vi "4 - Save a Well-Documented File (Solution).vi"() -> ()   [LabVIEW 2013]
uses:
  <vilib>/DAQmx/read.llb/DAQmx Read (Analog 1D Wfm NChan NSamp).vi
  <vilib>/DAQmx/miscellaneous.llb/DAQmx Fill In Error Info.vi
panel:
  out "Alarm Output":bool
  in  "Alarm Level":dbl=26.0
  out "Temperature":waveform(dbl)[](graph)
  in  "stop":bool
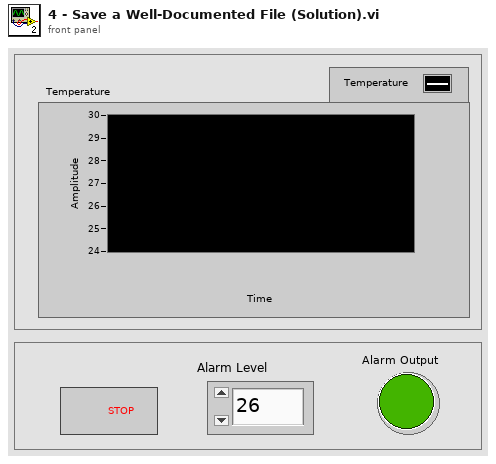
[diagram p1: front panel]
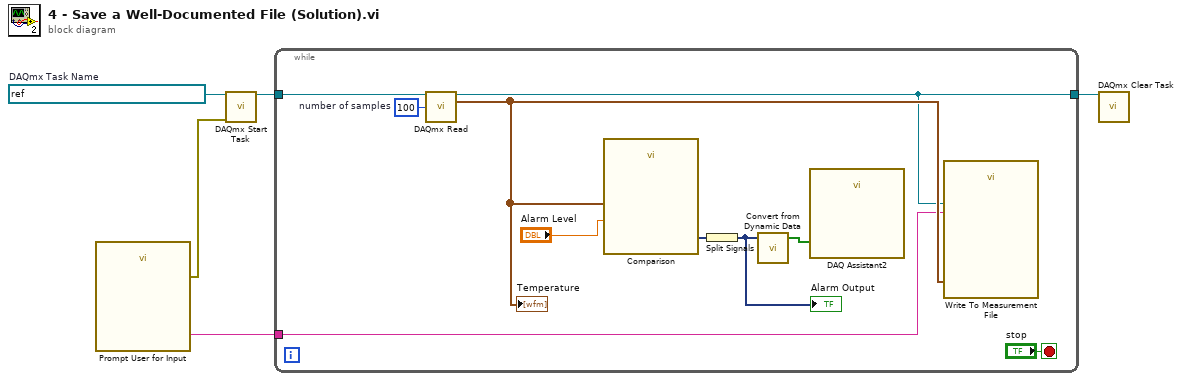
[diagram p0: block diagram]
diagram:
  w3 = refnum<k21> "Measure Temperature and Light"  # DAQmx Task Name
  n1 = call "Prompt User for Input"() -> ("Response"=w2:string, "error out"=w1:errorcluster)  [unwired: 17 in, 1 out]
  n2 = call <vilib>:"DAQmx Start Task.vi"("task/channels in"=w3, "error in"=w1) -> ("task out"=w5:refnum<k21>)  [unwired: 12 in, 1 out]
  n3 = while {
    tunnel: w5 -> [w11]
    tunnel: [w7] -> w4
    tunnel: w2 -> [w6]
    stop <- "stop" stop-if-true
    w9 = 100  # number of samples
    n4 = call-poly <vilib>:"DAQmx Read.vi"("task/channels in"=w11, "number of samples per channel"=w9) -> ("task out"=w7:refnum<k21>, "data"=w10:waveform(dbl)[])  [unwired: 11 in, 1 out]
    "Temperature" <- w10
    n5 = call "Comparison"("Operand 2"="Alarm Level", "Operand 1"=w10) -> ("Result"=w13:dynamicdata)  [unwired: 1 in, 8 out]
    n6 = Split Signals(w13) -> (w8:dynamicdata)  [unwired: 1 in]
    "Alarm Output" <- w8
    n7 = call "Convert from Dynamic Data"("Dynamic Data Type"=w8) -> ("Array"=w12:bool[])  [unwired: 3 in]
    n8 = call "DAQ Assistant2"("data"=w12) -> ()  [unwired: 4 in, 15 out]
    n9 = call "Write To Measurement File"("Signals"=w10, "Comment"=w6, "DAQmx Task"=w7) -> ()  [unwired: 14 in, 3 out]
  }
  n10 = call <vilib>:"DAQmx Clear Task.vi"("task in"=w4) -> ()  [unwired: 14 in, 1 out]
